vi "EF_InitQueuesAndEvents.vi"() -> (3 "EF_AllQRefs":T1, 5 "ExitRef":refnum<event-registration>, 7 "Exit":refnum<user-event>)   [LabVIEW 2017]
uses:
  Types/EF_AllQRefs.ctl
  Types/EF_GUIThread_QRef.ctl
  Types/EF_GUIThread_QData.ctl
  Types/EF_GUIThread_QCmds.ctl
  Types/EF_DAQThread_QRef.ctl
  Types/EF_DAQThread_QData.ctl
  Types/EF_DAQThread_QCmds.ctl
  Types/EF_DataProcThread_QRef.ctl
  Types/EF_DataProcThread_QData.ctl
  Types/EF_DataProcThread_QCmds.ctl
  Types/EF_AnalysisThread_QRef.ctl
  Types/EF_AnalysisThread_QData.ctl
  Types/EF_AnalysisThread_QCmds.ctl
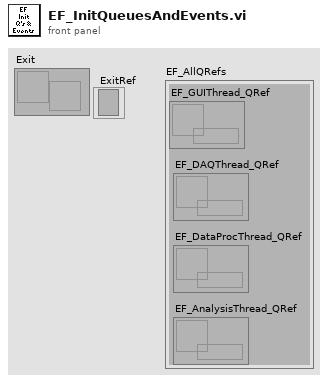
[diagram p1: front panel]
types:
  T1 = typedef "EF_AllQRefs.ctl" = cluster{"EF_GUIThread_QRef":T2, "EF_DAQThread_QRef":T3, "EF_DataProcThread_QRef":T4, "EF_AnalysisThread_QRef":T5}
  T2 = typedef "EF_GUIThread_QRef.ctl" = refnum<queue>
  T3 = typedef "EF_DAQThread_QRef.ctl" = refnum<queue>
  T4 = typedef "EF_DataProcThread_QRef.ctl" = refnum<queue>
  T5 = typedef "EF_AnalysisThread_QRef.ctl" = refnum<queue>
  T6 = typedef "EF_DataProcThread_QData.ctl" = cluster{"EF_DataProc_Cmds":T7, "nActual":i32, "Buffer":u32[], "TickCount":u32, "Param":i32}
  T7 = typedef "EF_DataProcThread_QCmds.ctl" = enum16{"Exit", "Proc", "Init", "SetShift", "SetThres"}
  T8 = typedef "EF_AnalysisThread_QData.ctl" = cluster{"Cmd":T9, "Histo":u32[], "DecayT0":dbl, "HistoRes":dbl, "TotalBinHistStart":u64, "TimeTraceRes":dbl, "Total bin":u64, "TickCount":u32, "LTThreshold":dbl, "TTLActivate":bool, "TTLDelay":dbl, "TTLWidth":dbl, "MinIntCounts":u32}
  T9 = typedef "EF_AnalysisThread_QCmds.ctl" = enum16{"Exit", "CalcAvgLT", "CalcDelay", "SetDecayT0", "SetHistoRes", "SetTimeTraceRes", "SetLTThreshold", "SetTTLActiv", "SetTTLDelay", "SetTTLWidth", "SetMinIntCounts"}
  T10 = typedef "EF_GUIThread_QData.ctl" = cluster{"Histo":u32[], "Rates":i32[], "Cmd":T11, "Res":dbl, "TimeTrace":u32[], "Bin":i32, "Status":string, "Total bin":u64, "AvgLTs":dbl[], "TotalBinsHistStart":u64[], "HistStartTimes":dbl[], "MinDelays":dbl[], "ShortDelay":bool, "Pending TTLs":i32, "error in (no error)":errorcluster, "DeltaT":dbl, "NumLTs":i32}
  T11 = typedef "EF_GUIThread_QCmds.ctl" = enum16{"_none_", "Res", "Histo", "TTrace", "Lifetime", "Rates", "Status", "ShortDelay", "_Error_"}
  T12 = typedef "EF_DAQThread_QData.ctl" = cluster{"EF_DAQThread_Cmds":T13, "Parameter":i32[], "error in (no error)":errorcluster}
  T13 = typedef "EF_DAQThread_QCmds.ctl" = enum16{"Idle", "Init", "InitHW", "SetCFD0", "SetCFD1", "SetCh0Divider", "SetCh0Offset", "SetOffset", "SetBinning", "GetResolution", "GetRates", "StartMeas", "ReadFiFo", "StopMeas", "WriteStatus", "_Error_", "Exit"}
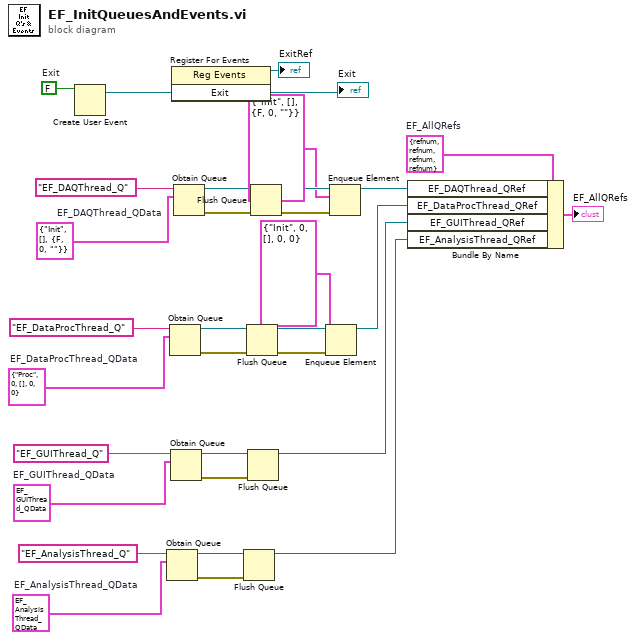
[diagram p0: block diagram]
diagram:
  w7 = T1 {"EF_GUIThread_QRef"=refnum, "EF_DAQThread_QRef"=refnum, "EF_DataProcThread_QRef"=refnum, "EF_AnalysisThread_QRef"=refnum}  # EF_AllQRefs
  w8 = T8 {"Cmd"=enum."Exit", "Histo"=[], "DecayT0"=0.0, "HistoRes"=0.0, "TotalBinHistStart"=0, "TimeTraceRes"=0.0, "Total bin"=0, "TickCount"=0, "LTThreshold"=0.0, "TTLActivate"=FALSE, "TTLDelay"=0.0, "TTLWidth"=0.0, "MinIntCounts"=0}  # EF_AnalysisThread_QData
  w12 = T10 {"Histo"=[], "Rates"=[], "Cmd"=enum."_none_", "Res"=0.0, "TimeTrace"=[], "Bin"=0, "Status"="", "Total bin"=0, "AvgLTs"=[], "TotalBinsHistStart"=[], "HistStartTimes"=[], "MinDelays"=[], "ShortDelay"=FALSE, "Pending TTLs"=0, "error in (no error)"={"status"=FALSE, "code"=0, "source"=""}, "DeltaT"=0.0, "NumLTs"=0}  # EF_GUIThread_QData
  w16 = T6 {"EF_DataProc_Cmds"=enum."Proc", "nActual"=0, "Buffer"=[], "TickCount"=0, "Param"=0}  # EF_DataProcThread_QData
  w24 = FALSE  # Exit
  w30 = T12 {"EF_DAQThread_Cmds"=enum."Init", "Parameter"=[], "error in (no error)"={"status"=FALSE, "code"=0, "source"=""}}  # EF_DAQThread_QData
  n1 = Create User Event(user event datatype=w24) -> (user event=w23:refnum<user-event>)  [unwired: 1 in, 1 out]
  "Exit" <- w23
  n2 = Obtain Queue(name (unnamed)="EF_AnalysisThread_Q", element data type=w8) -> (queue out=w11:refnum<queue>, error out=w10:errorcluster)  [unwired: 3 in, 1 out]
  n3 = Obtain Queue(name (unnamed)="EF_DataProcThread_Q", element data type=w16) -> (queue out=w21:refnum<queue>, error out=w18:errorcluster)  [unwired: 3 in, 1 out]
  n4 = Obtain Queue(name (unnamed)="EF_GUIThread_Q", element data type=w12) -> (queue out=w13:refnum<queue>, error out=w14:errorcluster)  [unwired: 3 in, 1 out]
  n5 = register-events(w23) -> (reference out=→"ExitRef":refnum<event-registration>)  [unwired: 2 in, 1 out]
  n6 = Obtain Queue(name (unnamed)="EF_DAQThread_Q", element data type=w30) -> (queue out=w25:refnum<queue>, error out=w29:errorcluster)  [unwired: 3 in, 1 out]
  n7 = Flush Queue(queue=w11, error in (no error)=w10) -> (queue out=w3:refnum<queue>)  [unwired: 2 out]
  n8 = Flush Queue(queue=w21, error in (no error)=w18) -> (queue out=w20:refnum<queue>, error out=w19:errorcluster)  [unwired: 1 out]
  n9 = Flush Queue(queue=w13, error in (no error)=w14) -> (queue out=w4:refnum<queue>)  [unwired: 2 out]
  n10 = Flush Queue(queue=w25, error in (no error)=w29) -> (queue out=w27:refnum<queue>, error out=w28:errorcluster)  [unwired: 1 out]
  n11 = Enqueue Element(queue=w20, element=T6 {"EF_DataProc_Cmds"=enum."Init", "nActual"=0, "Buffer"=[], "TickCount"=0, "Param"=0}, error in (no error)=w19) -> (queue out=w5:refnum<queue>)  [unwired: 1 in, 2 out]
  n12 = Enqueue Element(queue=w27, element=T12 {"EF_DAQThread_Cmds"=enum."Init", "Parameter"=[], "error in (no error)"={"status"=FALSE, "code"=0, "source"=""}}, error in (no error)=w28) -> (queue out=w6:refnum<queue>)  [unwired: 1 in, 2 out]
  n13 = Bundle By Name(cluster=w7, "EF_DAQThread_QRef"=w6, "EF_DataProcThread_QRef"=w5, "EF_GUIThread_QRef"=w4, "EF_AnalysisThread_QRef"=w3) -> (→"EF_AllQRefs":T1)
